vi "GetMetadata.vi"(7 "Msg":refnum<class "Msg.lvclass">) -> (3 "Metadata":T1 {"AbsoluteTime" format="%<%x %.3X>T"})   [LabVIEW 2020, in "_Template.lvlib" / "{{Msg}}.lvlib" / "Msg.lvclass"]
uses:
  Msg.lvclass
  jettl/jettl/Metadata/Metadata.lvclass
  Msg.lvclass/Msg.ctl
  jettl/jettl/Lifecycle.ctl
  jettl/jettl/jettl.lvlib
  jettl/jettl/Metadata.ctl
  jettl/jettl/Origin.ctl
panel:
  # "This front panel should not be manipulated."
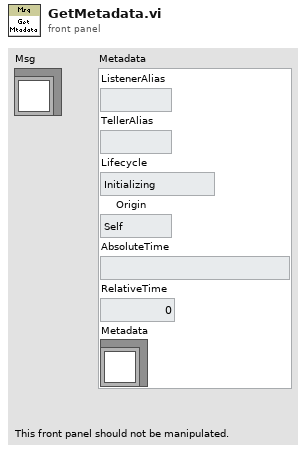
[diagram p1: front panel]
types:
  T1 = typedef "jettl.lvlib/Metadata.ctl" = cluster{"ListenerAlias":string, "TellerAlias":string, "Lifecycle":T2, "Origin":T3, "AbsoluteTime":timestamp, "RelativeTime":dbl, "Metadata":refnum<class "Metadata.lvclass">}
  T2 = typedef "jettl.lvlib/Lifecycle.ctl" = enum16{"Initializing", "SettingUp", "Starting", "Running", "Stopping", "TearingDown", "Terminated"}
  T3 = typedef "jettl.lvlib/Origin.ctl" = enum16{"Self", "Parent", "Child"}
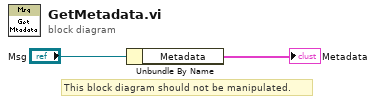
[diagram p0: block diagram]
diagram:
  # "This block diagram should not be manipulated."
  n1 = Unbundle By Name("Msg") -> ("Metadata"=→"Metadata":T1)
